vi "Read Local Context.vi"(8 "error in (no error)":errorcluster, 11 "Client Proxy LNA in":refnum<class "Client Proxy LNA.lvclass">) -> (0 "error out":errorcluster, 2 "Local Context":string, 3 "Client Proxy LNA out":refnum<class "Client Proxy LNA.lvclass">)   [LabVIEW 2026]
uses:
  Client Proxy LNA.lvclass
  C:/Users/E2013170/Documents/GitHub/Measurement-Utility-Reference/recovery/packages/ni_lib_linked_network_actor-1.2.0.19-9492AF5A82/File Group 0/vi.lib/NI/Actors/Linked Network Actor/Linked Network Actor/Linked Network Actor.lvclass
  C:/Program Files/National Instruments/LabVIEW 2026/vi.lib/ActorFramework/Actor/Actor.lvclass
  C:/Users/E2013170/Documents/GitHub/Measurement-Utility-Reference/components/HAL-MAL-Application/Source/Framework/Server/Client Proxy LNA/Client Proxy LNA.lvclass
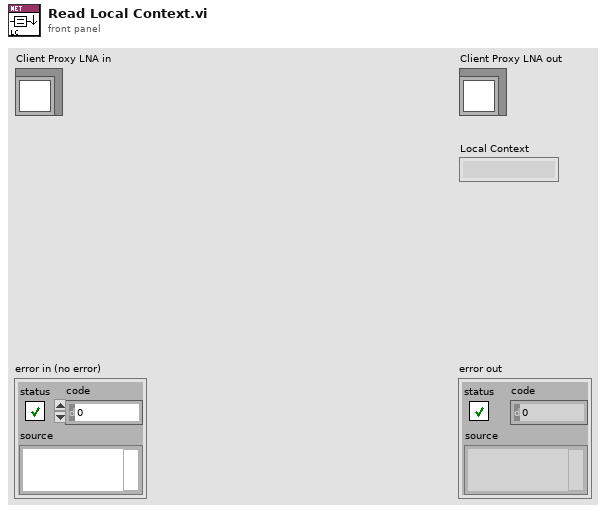
[diagram p1: front panel]
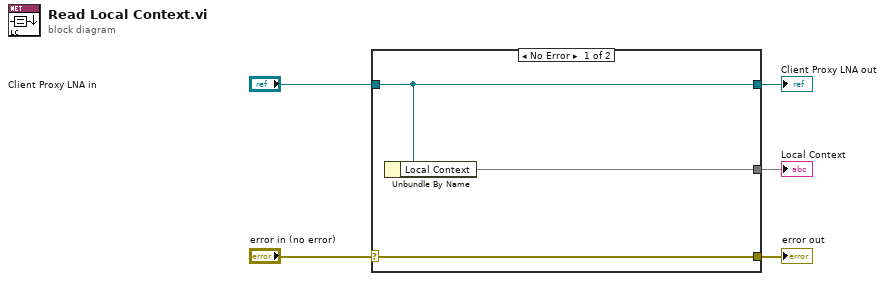
[diagram p0: block diagram]
diagram:
  n1 = case shown="No Error" "error in (no error)" {
    selector: "error in (no error)" -> [w8 w9]
    tunnel: [w8 w9] -> w4
    tunnel: [w7 w10] -> w2
    tunnel: "Client Proxy LNA in" -> [w7 w10]
    tunnel: [w6 _] -> w1
    frame No Error {
      n2 = Unbundle By Name(w7) -> ("Local Context"=w6)
    }
    frame Error {
    }
  }
  "error out" <- w4
  "Client Proxy LNA out" <- w2
  "Local Context" <- w1
